vi "Using_the_compass.vi"() -> ()   [LabVIEW 2009]
panel:
  in  "Location":u16(ring) items=["Virgina Beach", "School"]
  in  "stop":bool
  out "Turn rate":dbl
  out "Compass Data":T1={"Heading (deg)"=130.6, "Pitch (deg)"=-0.5, "Roll (deg)"=-0.7}
  in  "Compass Com Port":refnum<visa-resource-name>="COM4"
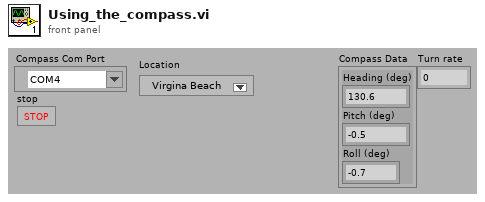
[diagram p1: front panel]
types:
  T1 = cluster{"Heading (deg)":dbl, "Pitch (deg)":dbl, "Roll (deg)":dbl}
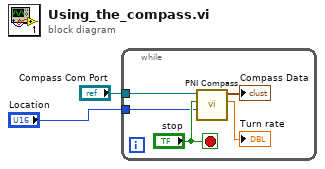
[diagram p0: block diagram]
diagram:
  n1 = while {
    tunnel: "Compass Com Port" -> [w7]
    tunnel: "Location" -> [w3]
    stop <- "stop" stop-if-true
    n2 = call "PNI Compass.vi"("Location"=w3, "Stop"="stop", "Compass Com Port"=w7) -> ("Turn rate"=→"Turn rate":dbl, "Compass Data"=→"Compass Data":T1)  [unwired: 7 in]
  }
